vi "Set Announce Interval.vi"(8 "error in (no error)":errorcluster, 10 "Announce Interval":dbl, 11 "Node in":refnum<class "Node.lvclass">) -> (0 "error out":errorcluster, 3 "Node out":refnum<class "Node.lvclass">)   [LabVIEW 2020, in "VolatusConfig.lvlib" / "Node.lvclass"]
uses:
  Node.lvclass
  Node.lvclass/Node.ctl
  VolatusConfigElement/VolatusConfigElement.lvclass
  lv-cdm/CDM-Config/Config Element/Config Element.lvclass
  C:/dev/lv20CE/relink/lv-volatus/VolatusConfig/VolatusConfigElement/VolatusConfigElement.lvclass
  C:/dev/lv20CE/relink/lv-volatus/VolatusConfig/Node/Node.lvclass
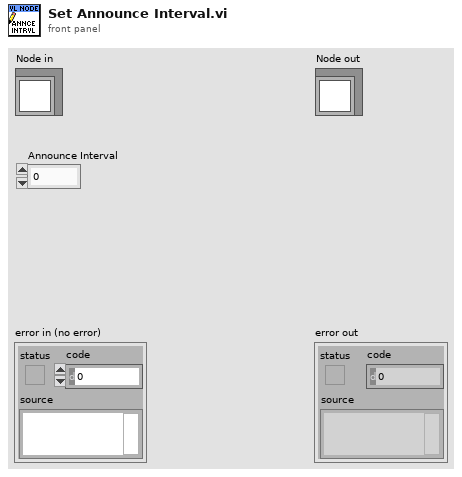
[diagram p1: front panel]
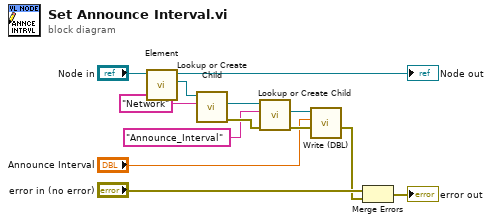
[diagram p0: block diagram]
diagram:
  n1 = call "Element.vi"("VolatusConfigElement in"="Node in") -> ("Element"=w11:refnum<class "Config Element.lvclass">, "VolatusConfigElement out"=→"Node out":refnum<class "Node.lvclass">)  [unwired: 9 in]
  n2 = call "Lookup or Create Child.vi"("Name"="Network", "Config Element in"=w11) -> ("error out"=w12:errorcluster, "Child"=w9:refnum<class "Config Element.lvclass">)  [unwired: 6 in, 2 out]
  n3 = call "Lookup or Create Child.vi"("error in (no error)"=w12, "Name"="Announce_Interval", "Config Element in"=w9) -> ("error out"=w4:errorcluster, "Child"=w5:refnum<class "Config Element.lvclass">)  [unwired: 5 in, 2 out]
  n4 = call "Write (DBL).vi"("error in (no error)"=w4, "DBL Value"="Announce Interval", "Config Element in"=w5) -> ("error out"=w1:errorcluster)  [unwired: 7 in, 1 out]
  n5 = Merge Errors("error in (no error)", w1) -> (→"error out":errorcluster)
